vi "Main.vi"(8 "error in (no error)":errorcluster, 11 "TemplateBase in":refnum<class "Template.lvclass">) -> (0 "error out":errorcluster, 3 "component":refnum<class "Template.lvclass">)   [LabVIEW 2012, in "Template.lvclass"]
doc: "Main VI of the component."
uses:
  Template.lvclass
  <vilib>/Distrio/Murmex/Murmex/command_enum.ctl
  <vilib>/Distrio/Murmex/InitialiseMessage/InitialiseMessage.lvclass
  <vilib>/Distrio/Murmex/TerminateMessage/TerminateMessage.lvclass
  <vilib>/Distrio/Murmex/ConfigureMessage/ConfigureMessage.lvclass
  <vilib>/Distrio/Murmex/Murmex/Set configure at initialise.vi
  <vilib>/Distrio/Murmex/Murmex/Set log reference.vi
  <vilib>/Distrio/Murmex/Murmex/Set VI reference.vi
  <vilib>/Distrio/Murmex/Murmex/Murmex.lvclass
  <vilib>/Distrio/Murmex/Message/Message.lvclass
panel:
  in  "button:configure":bool
  in  "generic command":string
  in  "button:send command":bool
  in  "command":T1
  in  "id":string
  in  "button:quit":bool
  out "terminate?":bool
  out "log":string
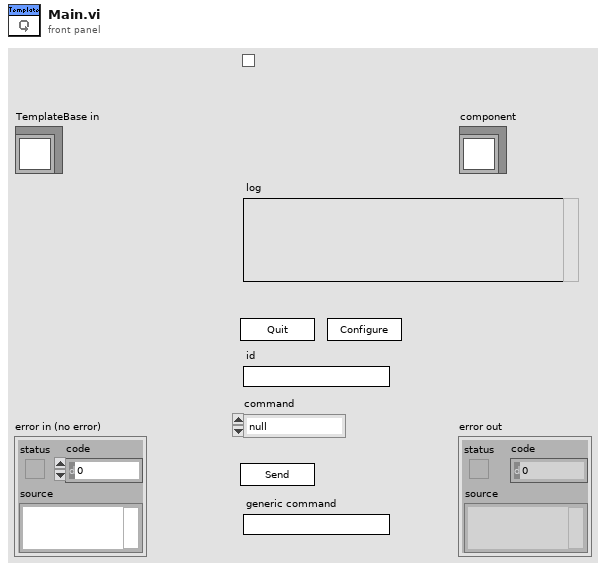
[diagram p1: front panel]
types:
  T1 = typedef "Murmex.lvlib/Murmex.lvclass/command_enum.ctl" = enum16{"null", "initialise", "reset", "terminate", "acknowledge", "update", "inspect", "inform", "proceed", "start", "stop", "fetch", "configure", "generic"}
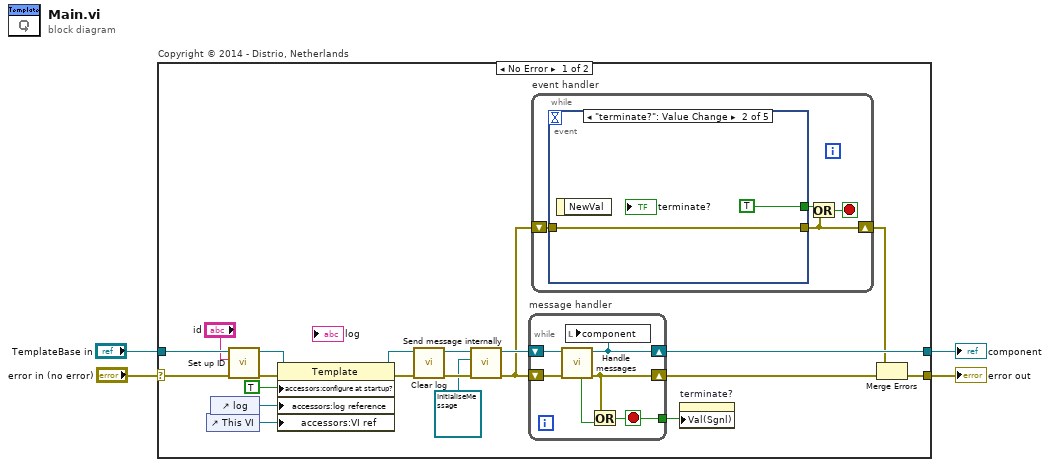
[diagram p0: block diagram]
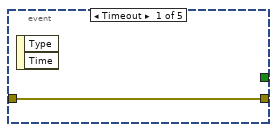
[diagram p2: hidden frame]
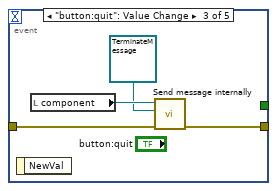
[diagram p3: hidden frame]
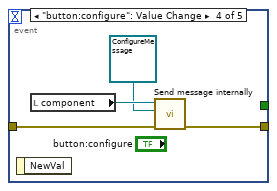
[diagram p4: hidden frame]
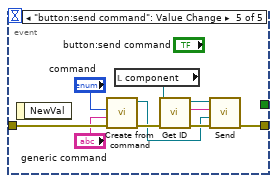
[diagram p5: hidden frame]
diagram:
  n1 = case "Copyright © 2014 - Distrio, Netherlands" shown="No Error" "error in (no error)" {
    selector: "error in (no error)" -> [w5 w57]
    tunnel: [w24 w56] -> w4
    tunnel: "TemplateBase in" -> [w11 w56]
    tunnel: [w6 w57] -> w2
    frame No Error {
      n2 = control-ref of="This VI"() -> (w20:refnum<vi>)
      n3 = control-ref of="log"() -> (w21:refnum<vi>)
      n4 = call <vilib>:"Set up ID.vi"("error in (no error)"=w5, "component ID"="id", "MurmexBase in"=w11) -> ("error out"=w12:errorcluster, "MurmexBase out"=w10:refnum<class "Template.lvclass">)  [unwired: 6 in, 1 out]
      n5 = property class="Template"(reference=w10, error in=w12, "accessors:configure at startup?"=TRUE ("configure at startup?"), "accessors:log reference"=w21, "accessors:VI ref"=w20) -> (reference out=w23:refnum<class "Template.lvclass">, error out=w17:errorcluster)
      n6 = call <vilib>:"Clear log.vi"("error in (no error)"=w17, "MurmexBase in"=w23) -> ("error out"=w16:errorcluster, "MurmexBase out"=w19:refnum<class "Template.lvclass">)  [unwired: 8 in]
      n7 = call <vilib>:"Send message internally.vi"("error in (no error)"=w16, "Message"=refnum<class "InitialiseMessage.lvclass"> refnum ("InitialiseMessage"), "Murmex in"=w19) -> ("error out"=w13:errorcluster, "Murmex out"=w18:refnum<class "Template.lvclass">)  [unwired: 7 in]
      n8 = while "message handler" {
        shift-right: [w53] -> w7
        shift-left: w13 -> [w55]
        shift-right: [w50] -> w24
        shift-left: w18 -> [w54]
        tunnel: [w51] -> w14
        stop <- w51 stop-if-true
        n9 = call <vilib>:"Handle messages.vi"("error in (no error)"=w55, "Murmex in"=w54) -> ("error out"=w53:errorcluster, "Murmex out"=w50:refnum<class "Template.lvclass">, "terminated?"=w52:bool)  [unwired: 7 in]
        n10 = local write "component"(w50) -> ()
        n11 = Or(x=w53, y=w52) -> (x .or. y?=w51:bool)
      }
      n12 = while "event handler" {
        shift-right: [w27] -> w8
        shift-left: w13 -> [w28]
        stop <- w25 stop-if-true
        n13 = event shown="[1] \"terminate?\": Value Change" {
          selector: _ -> [_ _ _ _ _]
          dyn-events: _ -> [_ _ _ _ _]
          timeout: _ -> [_ _ _ _ _]
          tunnel: w28 -> [w29 w31 w35 w39 w45]
          tunnel: [w29 w31 w33 w37 w42] -> w27
          tunnel: [_ TRUE _ _ _] -> w26
          event Timeout {
            n14 = event-data() -> ()  [unwired: 1 in, 2 out]
          }
          event "terminate?": Value Change {
            n15 = event-data() -> ()  [unwired: 1 in, 1 out]
          }
          event "button:quit": Value Change {
            n16 = event-data() -> ()  [unwired: 1 in, 1 out]
            n17 = local read "component"() -> (w34:refnum<class "Template.lvclass">)
            n18 = call <vilib>:"Send message internally.vi"("error in (no error)"=w35, "Message"=refnum<class "TerminateMessage.lvclass"> refnum ("TerminateMessage"), "Murmex in"=w34) -> ("error out"=w33:errorcluster)  [unwired: 7 in, 1 out]
          }
          event "button:configure": Value Change {
            n19 = event-data() -> ()  [unwired: 1 in, 1 out]
            n20 = local read "component"() -> (w38:refnum<class "Template.lvclass">)
            n21 = call <vilib>:"Send message internally.vi"("error in (no error)"=w39, "Message"=refnum<class "ConfigureMessage.lvclass"> refnum ("Distrio Murmex 1.5:ConfigureMessage"), "Murmex in"=w38) -> ("error out"=w37:errorcluster)  [unwired: 7 in, 1 out]
          }
          event "button:send command": Value Change {
            n22 = event-data() -> ()  [unwired: 1 in, 1 out]
            n23 = call <vilib>:"Create from command.vi"("error in (no error)"=w45, "generic command"="generic command", "command"="command") -> ("error out"=w44:errorcluster, "Message out"=w43:refnum<class "Message.lvclass">)  [unwired: 7 in]
            n24 = local read "component"() -> (w48:refnum<class "Template.lvclass">)
            n25 = call <vilib>:"Get ID.vi"("error in (no error)"=w44, "Murmex in"=w48) -> ("error out"=w46:errorcluster, "component id"=w47:string, "Murmex out"=w49:refnum<class "Template.lvclass">)  [unwired: 7 in]
            n26 = call <vilib>:"Send.vi"("error in (no error)"=w46, "Message"=w43, "recipient"=w47, "Murmex in"=w49) -> ("error out"=w42:errorcluster)  [unwired: 6 in, 1 out]
          }
        }
        n27 = Or(x=w26, y=w27) -> (x .or. y?=w25:bool)
      }
      n28 = property on="terminate?" class="Bool (strict)"("Val(Sgnl)"=w14) -> ()  [unwired: 2 in, 2 out]
      n29 = Merge Errors(w8, w7) -> (w6:errorcluster)
    }
    frame Error {
    }
  }
  "error out" <- w2
  "component" <- w4
